vi "Shutdown.vi"(8 "error in (no error)":errorcluster, 11 "Mode":T1) -> (0 "error out":errorcluster)   [LabVIEW 2015]
uses:
  Re-use Libraries/Minimal Actor Framework/Messaging/Message/Message.lvclass
  Global Actor API References.vi
  Main Controller Actor API.lvclass
  Actor/Remote Mode.ctl
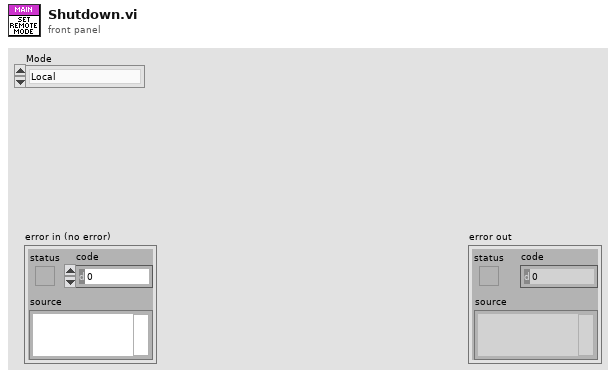
[diagram p1: front panel]
types:
  T1 = typedef "Main Controller Actor.lvclass/Remote Mode.ctl" = enum16{"Local", "Remote"}
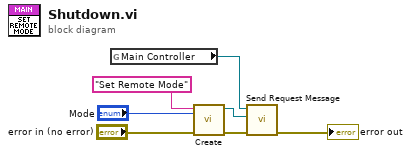
[diagram p0: block diagram]
diagram:
  n1 = global read "Global Actor API References.vi" "Main Controller"() -> (w3:refnum<class "Main Controller Actor API.lvclass">)
  n2 = call "Create.vi"("error in (no error)"="error in (no error)", "Data"="Mode", "Name"="Set Remote Mode" ("Parameter")) -> ("error out"=w4:errorcluster, "Message out"=w5:refnum<class "Message.lvclass">)  [unwired: 7 in]
  n3 = call-dynamic "Send Request Message.vi"("error in (no error)"=w4, "Message"=w5, "Actor API in"=w3) -> ("error out"=→"error out":errorcluster)  [unwired: 8 in]
